vi "Current Control Dakota.vi"(3 "AO0":i32(knob)=472 min=0 max=1023 scale=0.0..1023.0 scale format="%.2f") -> ()   [LabVIEW 2015]
uses:
  <vilib>/rvi/Emulation/niFpgaGetClockAttributes.vi
  <vilib>/rvi/Emulation/niFpgaSctlEmulationGetInTimedLoop.vi
  <vilib>/rvi/Emulation/niFpgaEmulationReportErrorSimple.vi
  <vilib>/rvi/eio/common/nirviEmuTemplateMethod_errors.vi
  <vilib>/rvi/interface/RandomDataEmulation/niFpgaRandomDataHandleErrors.vi
  <vilib>/rvi/Emulation/niFpgaCriticalErrorInLSC.vi
  <vilib>/eio/EIONode/EIONode.xnode
  <vilib>/rvi/DataTransferAndStorage/Container/XNode/niFpgaContainer.xnode
  <vilib>/rvi/interface/RandomDataEmulation/nirviRandomDataFpgaReadWriteTemplate.vi
panel:
  in  "Outlet Count(uSec)":i32 caption="Count(uSec)"
  out "Outlet Overflow?":bool
  in  "AO1":i32(knob)=405 min=198 max=1023 scale=198.0..1023.0 scale format="%.2f"
  in  "Inlet Count(uSec)":i32 caption="Count(uSec)"
  out "Inlet Overflow?":bool
  # "Overview\n======\n\nThis demonstrates how to control the PSV105 Valve. At 0 bits, the voltage across the 250 ohms, 30W resistor is 1.3V. This corresponds to 5.2mA, a little above the required current to turn the valve on according to the manufacturer. At 910 bits, we obtain a voltage of 5V across the shunt resistor; this corresponds to 20mA. \n\nConnection Protocols\n===============\nWire the AO0 pin on the C connector of the myRIo to the pin 3 of the non-inverting input of the opamp. Connect the power supplies andfollow the following instructions:\n\nInstructions:\n1.        Operate at constant pressure of 30 psi to get best results\n2.        Operate this valve between the DAC resolutions of 0 and  717 only. If you operate outside of this range, you might damage the valve.\n3.        Run the VI."
  # "Pin 14 Circuit"
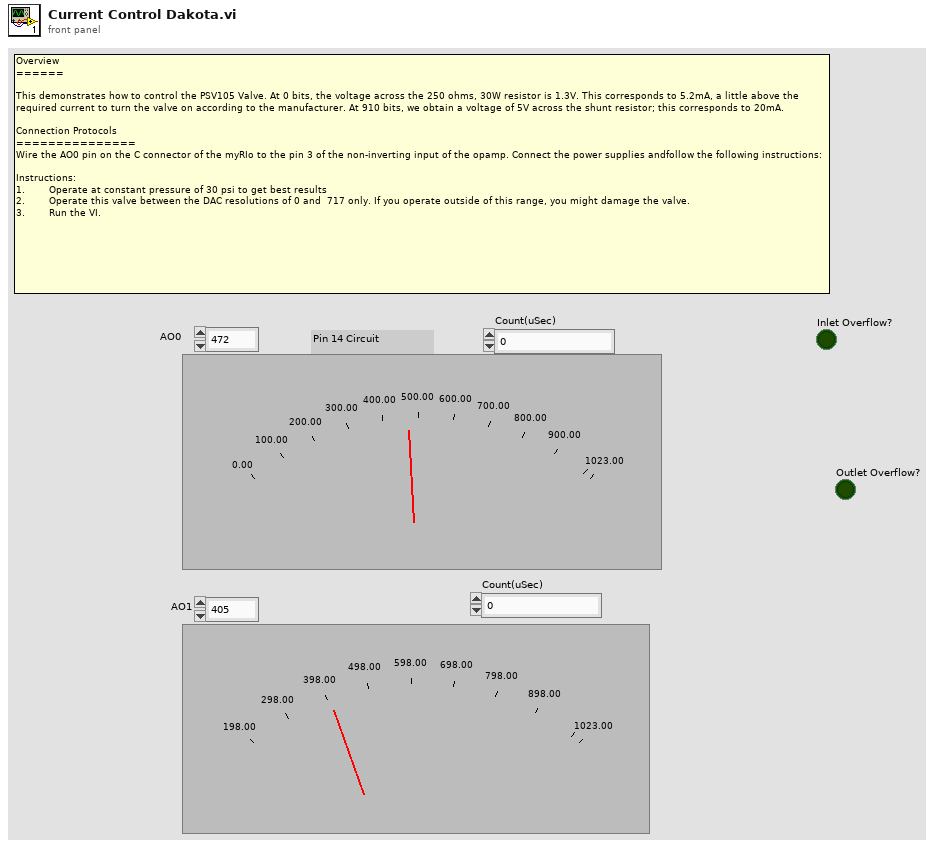
[diagram p1: front panel]
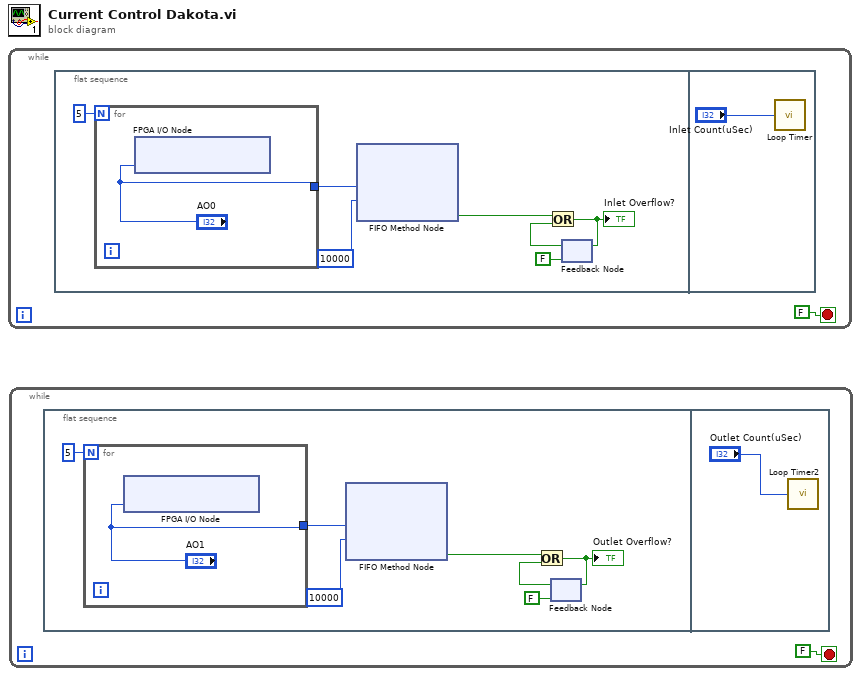
[diagram p0: block diagram]
diagram:
  n1 = while {
    stop <- FALSE stop-if-true
    n2 = flat-sequence {
      frame #0 {
        n3 = for {
          N: 5 -> [_]
          tunnel: ["AO0"] -> w3
          n4 = xnode "FPGA I/O Node"("ConnectorC/AO0"="AO0") -> ()  [unwired: 1 in, 1 out]
        }
        n5 = xnode ("FIFO Method Node")("Element"=w3, "Timeout"=10000) -> ("Timed Out?"=w5:bool)  [unwired: 1 in, 1 out]
        n6 = feedback #1(FALSE) -> (w7:bool)
        n7 = Or(x=w5, y=w7) -> (x .or. y?=w8:bool)
        "Inlet Overflow?" <- w8
        n8 = feedback-in #1(w8) -> ()
      }
      frame #1 {
        n9 = call "Loop Timer"("Count(uSec)"="Inlet Count(uSec)") -> ()  [unwired: 1 out]
      }
    }
  }
  n10 = while {
    stop <- FALSE stop-if-true
    n11 = flat-sequence {
      frame #0 {
        n12 = for {
          N: 5 -> [_]
          tunnel: ["AO1"] -> w13
          n13 = xnode "FPGA I/O Node"("ConnectorC/AO1"="AO1") -> ()  [unwired: 1 in, 1 out]
        }
        n14 = xnode ("FIFO Method Node")("Element"=w13, "Timeout"=10000) -> ("Timed Out?"=w15:bool)  [unwired: 1 in, 1 out]
        n15 = feedback #2(FALSE) -> (w17:bool)
        n16 = Or(x=w15, y=w17) -> (x .or. y?=w18:bool)
        "Outlet Overflow?" <- w18
        n17 = feedback-in #2(w18) -> ()
      }
      frame #1 {
        n18 = call "Loop Timer2"("Count(uSec)"="Outlet Count(uSec)") -> ()  [unwired: 1 out]
      }
    }
  }
